vi "FieldTheBall.vi"(4 "isOmni":bool, 6 "ReInit":bool, 11 "Original":T1) -> (2 "Ty":dbl format="%.2f", 3 "Tx":dbl format="%.2f")   [LabVIEW 2013]
uses:
  <vilib>/addons/control/pid/NI_PID_pid.lvlib
  <vilib>/addons/control/pid/pid.llb/PID (DBL).vi
  Common Code/Goal Info.ctl
  Common Code/Vision Packet.ctl
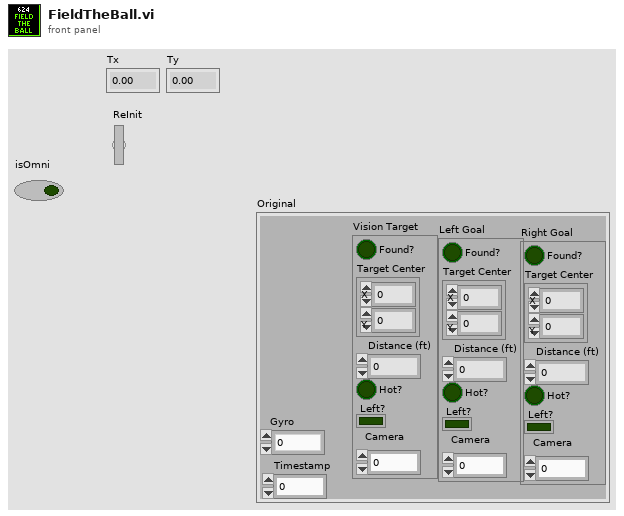
[diagram p1: front panel]
types:
  T1 = typedef "Vision Packet.ctl" = cluster{"Gyro":dbl, "Vision Target":T2, "Timestamp":u32, "Left Goal":T2, "Right Goal":T2}
  T2 = typedef "Goal Info.ctl" = cluster{"Found?":bool, "Target Center":cluster{"X":dbl, "Y":dbl}, "Distance (ft)":dbl, "Hot?":bool, "Left?":bool, "Camera":i16}
  T3 = cluster{"proportional gain (Kc)":dbl, "integral time (Ti, min)":dbl, "derivative time (Td, min)":dbl}
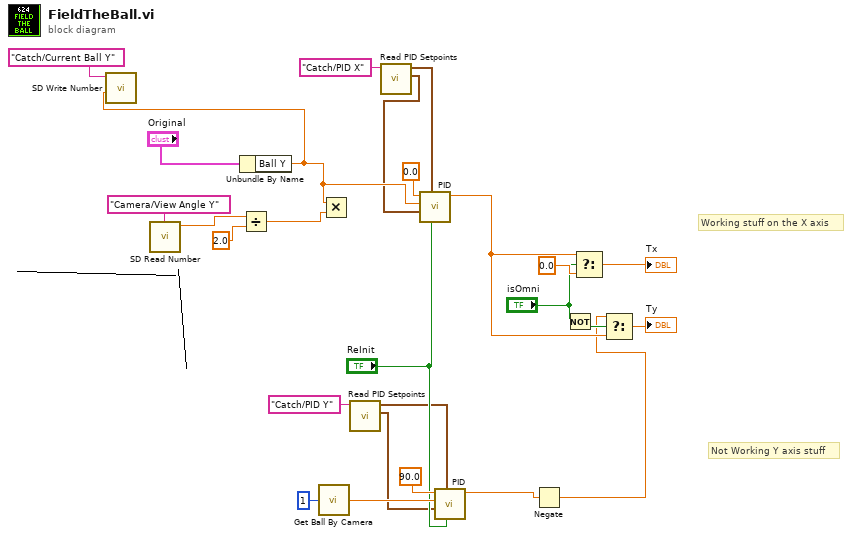
[diagram p0: block diagram]
diagram:
  # "Not Working Y axis stuff"
  # "Working stuff on the X axis"
  n1 = call <vilib>:"SD Read Number.vi"("Name"="Camera/View Angle Y") -> ("Numeric"=w25:dbl)  [unwired: 8 in, 2 out]
  n2 = Unbundle By Name("Original") -> ("Ball Y"=w14:dbl)
  n3 = call <vilib>:"SD Write Number.vi"("Numeric"=w14, "Name"="Catch/Current Ball Y") -> ()  [unwired: 8 in, 2 out]
  n4 = Divide(x=w25, y=2.0) -> (x/y=w23:dbl)
  n5 = call "Get Ball By Camera.vi"("Camera"=i16 1) -> ("Robot Relative Y"=w11:dbl)  [unwired: 9 in, 5 out]
  n6 = Multiply(x=w14, y=w23) -> ()  [unwired: 1 out]
  n7 = call "Read PID Setpoints.vi"("SD Name"="Catch/PID Y") -> ("PID gains"=w2:T3, "output range"=w3:cluster{"output high":dbl, "output low":dbl})  [unwired: 9 in]
  n8 = call "Read PID Setpoints.vi"("SD Name"="Catch/PID X") -> ("PID gains"=w5:T3, "output range"=w6:cluster{"output high":dbl, "output low":dbl})  [unwired: 9 in]
  n9 = call-poly <vilib>:"PID.vi"("reinitialize? (F)"="ReInit", "output range"=w6, "PID gains"=w5, "process variable"=w14, "setpoint"=0.0) -> ("output"=w20:dbl)  [unwired: 5 in, 1 out]
  n10 = call-poly <vilib>:"PID.vi"("reinitialize? (F)"="ReInit", "output range"=w3, "PID gains"=w2, "process variable"=w11, "setpoint"=90.0) -> ("output"=w10:dbl)  [unwired: 5 in, 1 out]
  n11 = Negate(x=w10) -> (-x=w9:dbl)
  n12 = Not(x="isOmni") -> (.not. x?=w12:bool)
  n13 = Select(t=w20, s="isOmni", f=0.0) -> (s? t:f=→"Tx":dbl)
  n14 = Select(t=w9, s=w12, f=w20) -> (s? t:f=→"Ty":dbl)
